vi "CRDS_Host_Test.vi"() -> ()   [LabVIEW 2012]
doc: "Host interface for communication with CRD and PAS. This application currently must be running before the servers (PAS and CRD chassis) are running). At startup, the host will poll the LAN for a UDP connection to each instrument, pinging on port 5555. The acquisition loop will configure the FP and then move into a waiting state where it is polling for a connection on TCP/IP using the STM Connection Manager. When one of the instruments responds to the host, a new TCP connection will be opened on port 5556 and added to the connection manager. Seeing the connection, this VI will move from a wait state to the acquisition state where connections will be monitored. \n\nDuring the acquisition state, the host will handle messages sent via TCP/IP from the instruments. A queued state machine will determine how the data packets sent from the different instruments is handled."
uses:
  Controls/rt_host_state.ctl
  <vilib>/Utility/Variable/NI_VariableUtilities.lvlib
  Controls/pasLasCtl.ctl
  Reusable/PAS/Main/Controls/Laser Modulation.ctl
  Utilities/FPGA/Controls/FPGAConfig.ctl
panel:
  in  "swDispl":T1
  in  "tabCtl":T2(tab)=enum."PAS Ctl"
  out "P":cluster{"hum":sgl, "dry":sgl, "ref":sgl} caption="Pressure (mb)" {"ref" format="%#.2f"; "dry" format="%#.2f"; "hum" format="%#.2f"}
  out "vaisalaData":T3 caption="Vaisala Data" {"ref"."TRH" format="%#.2f"; "ref"."RH" format="%#.2f"; "dry"."TRH" format="%#_2f"; "dry"."RH" format="%#_2f"; "hum"."TRH" format="%#_2g"; "hum"."RH" format="%#_2g"}
  out "alctData":T4 caption="Alicat Data" {"purge"."P" format="%.2f"; "purge"."T" format="%.2f"; "purge"."Q" format="%.2f"; "ref"."P" format="%.2f"; "ref"."T" format="%.2f"; "ref"."Q" format="%.2f"; "dry"."P" format="%.2f"; "dry"."T" format="%.2f"; "dry"."Q" format="%.2f"; "hum"."P" format="%.2f"; "hum"."T" format="%.2f"; "hum"."Q" format="%.2f"}
  in  "Laser Controls":cluster{"f (Hz)":dbl, "Duty Cycle (%)":dbl}
  in  "crdHeaterSP":cluster{"T1":sgl, "T2":sgl} caption="Heater Setpoints (degC)" {"T2" format="%.1f"; "T1" format="%.1f"}
  out "crdHeater":cluster{"T1":sgl, "T2":sgl} caption="Heater Temperature (degC)" {"T2" format="%.1g"; "T1" format="%.1g"}
  in  "crdFlows":T5 caption="Flow Rate Setpoints (LPM)" {"purge" max=5 format="%.2f"; "ref" max=5 format="%.2f"; "dry" max=5 format="%.2f"; "hum" max=5 format="%.2f"}
  out "crdTtec":sgl caption="TEC Temperature\n(degC)" format="%#.1f"
  in  "pasTECEn":T6 caption="Enable TECs"
  in  "pasTcell":T7 caption="Temperature \n (degC)"
  in  "pasFlows":T8 caption="Flow Rate Setpoint (LPM)" {"Cell 5" min=0.0 max=5.0; "Cell 4" min=0.0 max=5.0; "Cell 3" min=0.0 max=5.0; "Cell 2" min=0.0 max=5.0; "Cell 1" min=0.0 max=5.0}
  in  "pasLasCtl":T9={"Laser Output"={"Span"={"ch 1"=1.5, "ch 2"=1.5, "ch 3"=5.0, "ch 4"=5.0, "ch 5"=5.0}, "mod"={"ch 1"=enum."Sine", "ch 2"=enum."Sine", "ch 3"=enum."Sine", "ch 4"=enum."Sine", "ch 5"=enum."Sine"}}, "f0"={"Cell 1"=1360.2863, "Cell 2"=1358.2849, "Cell 3"=1355.6958, "Cell 4"=1355.4038, "Cell 5"=1352.1854}, "drive"=FALSE, "lasSysPow"=TRUE, "Speake Voltage"=0.0} caption="Laser Control" {"Laser Output"."Span"."ch 5" min=0 max=20; "Laser Output"."Span"."ch 4" min=0 max=20; "Laser Output"."Span"."ch 3" min=0 max=20; "Laser Output"."Span"."ch 2" min=0 max=20; "Laser Output"."Span"."ch 1" min=0 max=20; "f0"."Cell 1" format="%#.2f"; "f0"."Cell 2" format="%#.2f"; "f0"."Cell 3" format="%#.2f"; "f0"."Cell 4" format="%#.2f"; "f0"."Cell 5" format="%#.2f"}
  in  "DCPS":bool caption="DC Power Supply"
  in  "pasTteSP":sgl caption="TEC Temperature \nSetpoint (degC)" format="%#.2f"
  out "crdData":bool caption="CRD Data"
  out "pasErr":bool caption="PAS Error"
  out "pasCfg":bool caption="PAS Config"
  out "crdError":bool caption="CRDS Error"
  out "servAct":bool caption="Server Active"
  # "CRD Controls"
  # "CRD Controller Data"
  # "PAS Controls"
  # "PAS Housekeeping Data"
  # "TEC Temperature Control"
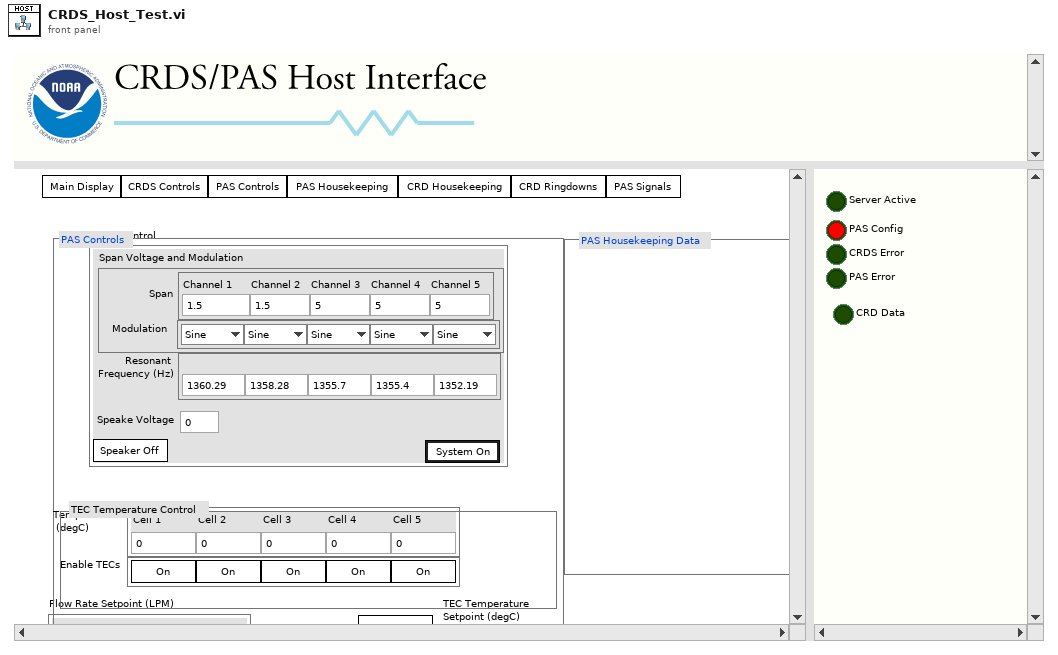
[diagram p1: front panel]
types:
  T1 = cluster{"mDispl":bool, "crdCtl":bool, "pasCtl":bool, "pasHK":bool, "crdHK":bool, "crdRD":bool, "pasSig":bool}
  T2 = enum32{"main", "CRDCtl", "PAS Ctl", "pasHK", "crdHK", "crdRD", "pasSig"}
  T3 = cluster{"hum":cluster{"RH":sgl, "TRH":sgl}, "dry":cluster{"RH":sgl, "TRH":sgl}, "ref":cluster{"RH":sgl, "TRH":sgl}}
  T4 = cluster{"hum":cluster{"Q":sgl, "T":sgl, "P":sgl}, "dry":cluster{"Q":sgl, "T":sgl, "P":sgl}, "ref":cluster{"Q":sgl, "T":sgl, "P":sgl}, "purge":cluster{"Q":sgl, "T":sgl, "P":sgl}}
  T5 = cluster{"hum":sgl, "dry":sgl, "ref":sgl, "purge":sgl}
  T6 = cluster{"Cell 1":bool, "Cell 2":bool, "Cell 3":bool, "Cell 4":bool, "Cell 5":bool}
  T7 = cluster{"Cell 1":sgl, "Cell 2":sgl, "Cell 3":sgl, "Cell 4":sgl, "Cell 5":sgl}
  T8 = cluster{"Cell 1":dbl, "Cell 2":dbl, "Cell 3":dbl, "Cell 4":dbl, "Cell 5":dbl}
  T9 = typedef "pasLasCtl.ctl" = cluster{"Laser Output":T10, "f0":cluster{"Cell 1":sgl, "Cell 2":sgl, "Cell 3":sgl, "Cell 4":sgl, "Cell 5":sgl}, "drive":bool, "lasSysPow":bool, "Speake Voltage":dbl}
  T10 = typedef "FPGAConfig.ctl" = cluster{"Span":cluster{"ch 1":sgl, "ch 2":sgl, "ch 3":sgl, "ch 4":sgl, "ch 5":sgl}, "mod":cluster{"ch 1":T11, "ch 2":T11, "ch 3":T11, "ch 4":T11, "ch 5":T11}}
  T11 = typedef "Laser Modulation.ctl" = enum8{"Sine", "Square"}
  T12 = typedef "rt_host_state.ctl" = enum16{"Config", "CRD Comm", "PAS Comm", "Wait", "Quit"}
  T13 = cluster{"c 1":bool, "c 2":bool, "c 3":bool, "c 4":bool, "c 5":bool}
  T14 = cluster{"[0]":bool, "[1]":bool, "[2]":bool, "[3]":bool, "[4]":bool, "[5]":bool, "[6]":bool}
  T15 = enum32{"invalid app kind", "Development System", "Run Time System", "Student Edition", "Embedded LabVIEW", "Evaluation", "Custom"}
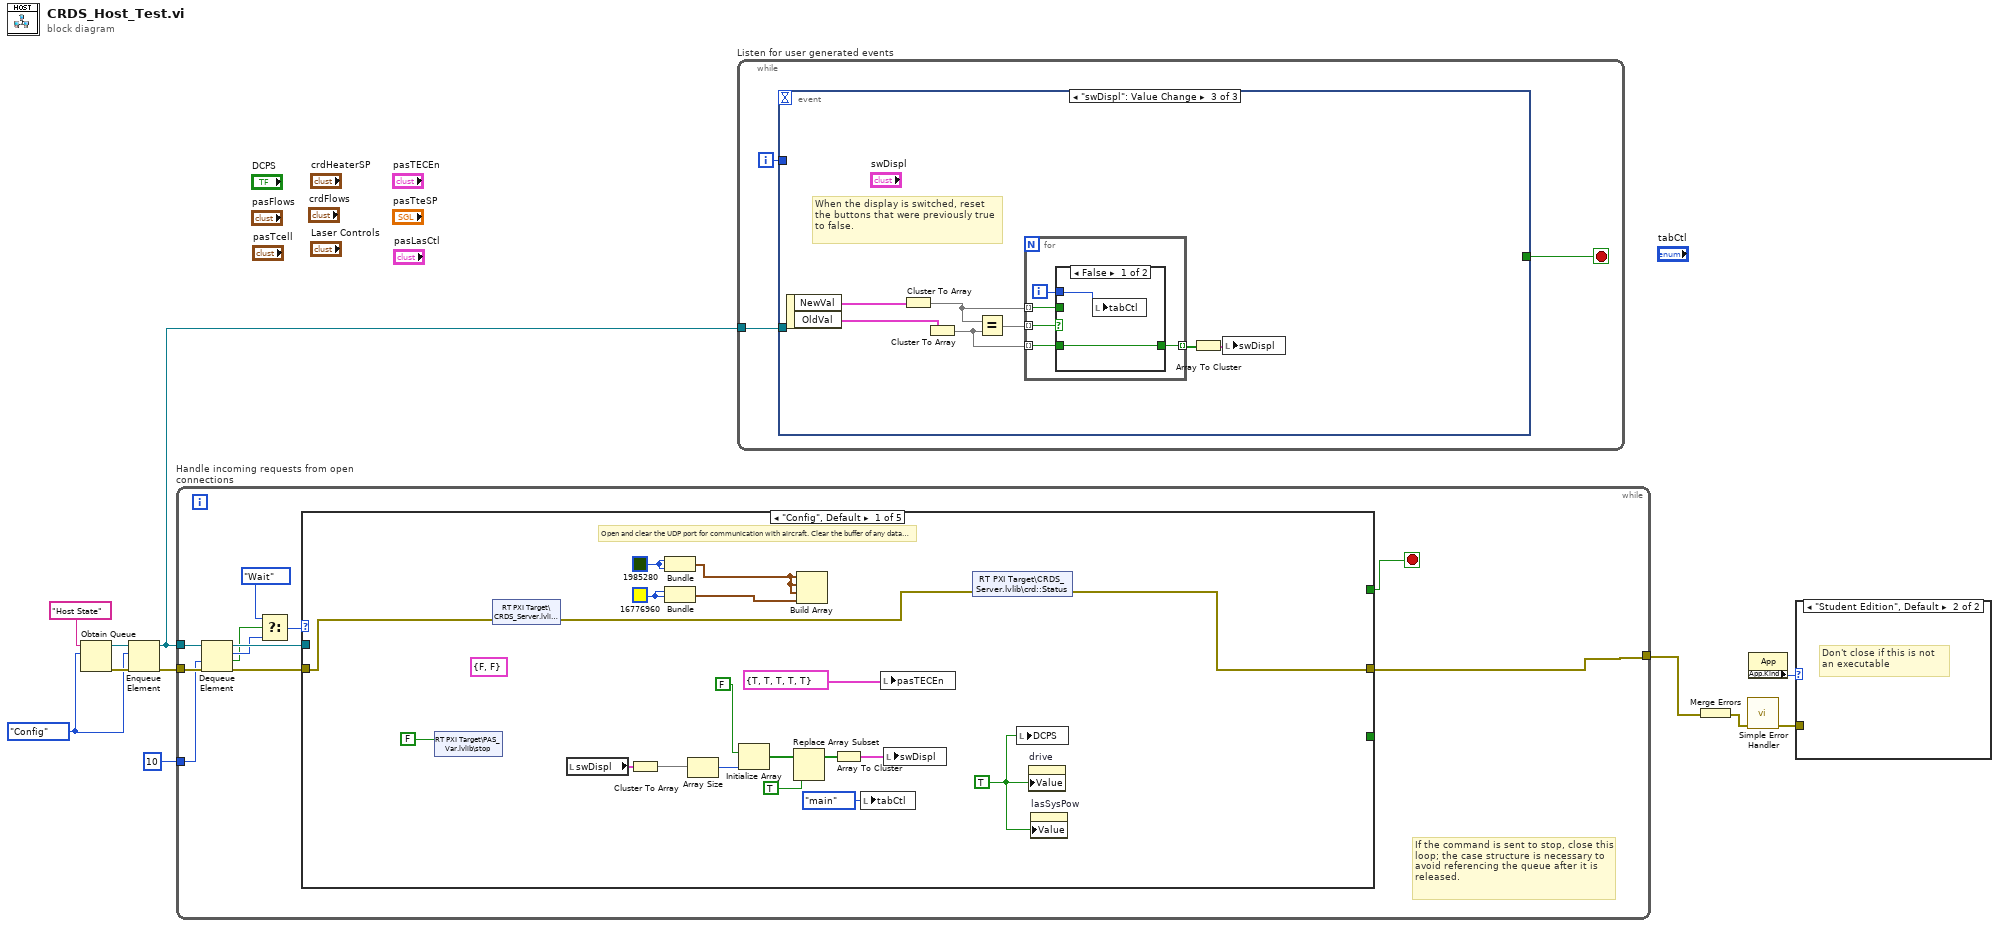
[diagram p0: block diagram]
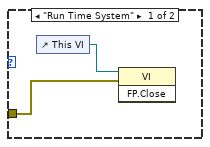
[diagram p2: hidden frame]
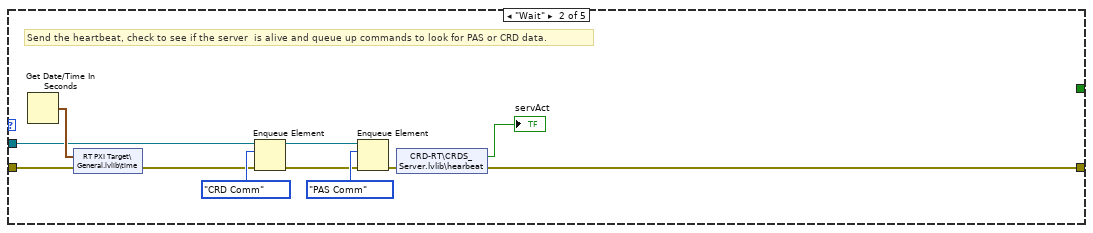
[diagram p3: hidden frame]
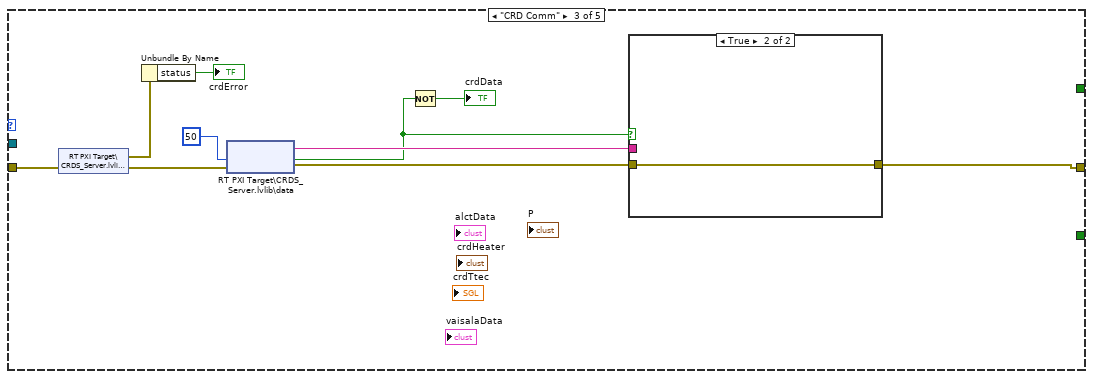
[diagram p4: hidden frame]
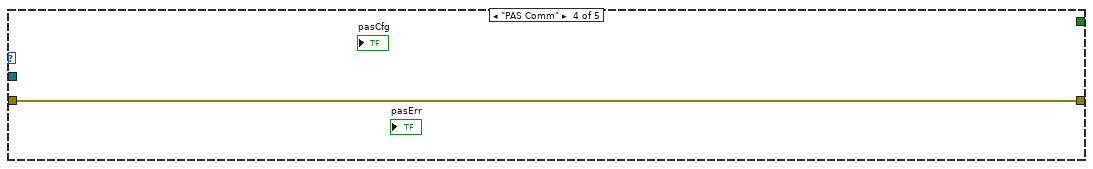
[diagram p6: hidden frame]
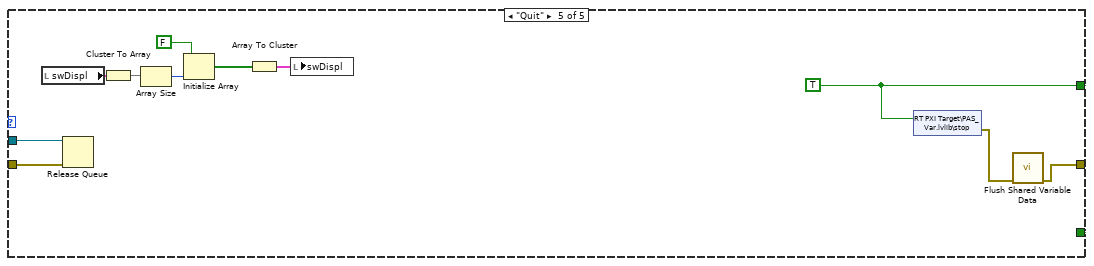
[diagram p7: hidden frame]
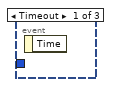
[diagram p8: hidden frame]
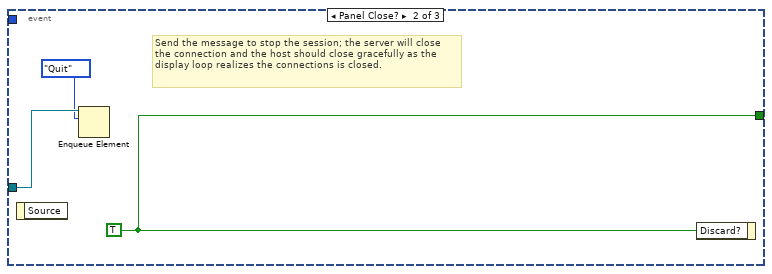
[diagram p9: hidden frame]
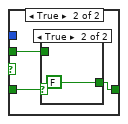
[diagram p10: hidden frame]
diagram:
  w7 = rt_host_state."Config" ("Host_State")
  n1 = Obtain Queue(name (unnamed)="Host State", element data type=w7) -> (queue out=w10:refnum<queue>, error out=w9:errorcluster)  [unwired: 3 in, 1 out]
  n2 = Enqueue Element(queue=w10, element=w7, error in (no error)=w9) -> (queue out=w1:refnum<queue>, error out=w8:errorcluster)  [unwired: 1 in, 1 out]
  n3 = while "Handle incoming requests from open connections" {
    tunnel: w1 -> [w22]
    tunnel: w8 -> [w20]
    tunnel: [w12] -> w6
    tunnel: 10 ("timeout in ms (-1)") -> [w13]
    stop <- w18 stop-if-true
    # "If the command is sent to stop, close this loop; the case structure is necessary to avoid referencing the queue after it is released."
    n4 = Dequeue Element(queue=w22, timeout in ms (-1)=w13, error in (no error)=w20) -> (queue out=w21:refnum<queue>, element=w17:T12, timed out?=w15:bool, error out=w19:errorcluster)
    n5 = Select(t=rt_host_state."Wait", s=w15, f=w17) -> (s? t:f=w14:T12)
    n6 = case shown="\"Config\", Default" w14 {
      tunnel: w19 -> [w24 w51 w58 w65 w69]
      tunnel: w21 -> [_ w50 _ _ w76]
      tunnel: [_ _ _ _ w68] -> w18
      tunnel: [_ _ _ _ w68] -> _
      tunnel: [w25 w49 w59 w65 w66] -> w12
      frame "Config", Default {
        w27 = TRUE ("Value")
        w29 = u32 16776960
        w28 = u32 1985280
        (unwired) cluster{"CRD":bool, "PAS":bool} {"CRD"=FALSE, "PAS"=FALSE} ("filtSwitch")
        # "Open and clear the UDP port for communication with aircraft. Clear the buffer of any data currently on line."
        n7 = shared-variable "RT PXI Target\\PAS_Var.lvlib\\stop"(FALSE ("stop")) -> ()  [unwired: 1 in, 1 out]
        n8 = shared-variable "RT PXI Target\\CRDS_Server.lvlib\\data"(error in=w24) -> (error out=w23:errorcluster)  [unwired: 1 out]
        n9 = local read "swDispl"() -> (w41:T1)
        n10 = Cluster To Array(cluster=w41) -> (array=w40:bool[])
        n11 = Bundle(w28, w28) -> (w31:cluster{u32, u32})  [unwired: 1 in]
        n12 = Bundle(w29, w29) -> (w30:cluster{u32, u32})  [unwired: 1 in]
        n13 = Array Size(array=w40) -> (size(s)=w39:i32)
        n14 = Initialize Array(FALSE, w39) -> (w38:bool[])
        n15 = Replace Array Subset(array=w38, new element=TRUE ("new element/subarray")) -> (w36:bool[])  [unwired: 1 in]
        n16 = Build Array(w31, w31, w31, w30) -> ()  [unwired: 1 out]
        n17 = Array To Cluster(array=w36) -> (cluster=w35:T14)
        n18 = local write "tabCtl"(T2."main" ("tabCtl")) -> ()
        n19 = local write "pasTECEn"(T13 {"c 1"=TRUE, "c 2"=TRUE, "c 3"=TRUE, "c 4"=TRUE, "c 5"=TRUE} ("pasTECEn")) -> ()
        n20 = local write "swDispl"(w35) -> ()
        n21 = shared-variable "RT PXI Target\\CRDS_Server.lvlib\\crd::Status"(error in=w23) -> (error out=w25:errorcluster)  [unwired: 1 out]
        n22 = local write "DCPS"(w27) -> ()
        n23 = property on="drive" class="Bool (strict)"("Value"=w27) -> ()  [unwired: 2 in, 2 out]
        n24 = property on="lasSysPow" class="Bool (strict)"("Value"=w27) -> ()  [unwired: 2 in, 2 out]
      }
      frame "Wait" {
        # "Send the heartbeat, check to see if the server  is alive and queue up commands to look for PAS or CRD data."
        n25 = Get Date/Time In Seconds() -> (seconds since 1Jan1904=w52:timestamp)
        n26 = shared-variable "RT PXI Target\\General.lvlib\\time"(w52, error in=w51) -> (error out=w42:errorcluster)
        n27 = Enqueue Element(queue=w50, element=rt_host_state."CRD Comm", error in (no error)=w42) -> (queue out=w47:refnum<queue>, error out=w43:errorcluster)  [unwired: 1 in, 1 out]
        n28 = Enqueue Element(queue=w47, element=rt_host_state."PAS Comm", error in (no error)=w43) -> (error out=w46:errorcluster)  [unwired: 1 in, 2 out]
        n29 = shared-variable "CRD-RT\\CRDS_Server.lvlib\\hearbeat"(error in=w46) -> (→"servAct":bool, error out=w49:errorcluster)
      }
      frame "CRD Comm" {
        n30 = shared-variable "RT PXI Target\\CRDS_Server.lvlib\\error"(error in=w58) -> (w56:errorcluster, error out=w57:errorcluster)
        n31 = Unbundle By Name(w56) -> ("status"=→"crdError":bool)
        n32 = shared-variable "RT PXI Target\\CRDS_Server.lvlib\\data"(error in=w57, 50 ("ms timeout (0)")) -> (w62:string, error out=w61:errorcluster, w54:bool)
        n33 = Not(x=w54) -> (.not. x?=→"crdData":bool)
        n34 = case shown="True" w54 {
          tunnel: w62 -> [_ _]
          tunnel: w61 -> [w63 w64]
          tunnel: [w63 w64] -> w59
          frame False {
          }
          frame True {
          }
        }
      }
      frame "PAS Comm" {
      }
      frame "Quit" {
        w68 = TRUE
        n35 = local read "swDispl"() -> (w75:T1)
        n36 = Release Queue(queue=w76, error in (no error)=w69) -> ()  [unwired: 1 in, 3 out]
        n37 = Cluster To Array(cluster=w75) -> (array=w74:bool[])
        n38 = Array Size(array=w74) -> (size(s)=w73:i32)
        n39 = Initialize Array(FALSE, w73) -> (w71:bool[])
        n40 = Array To Cluster(array=w71) -> (cluster=w70:T14)
        n41 = local write "swDispl"(w70) -> ()
        n42 = shared-variable "RT PXI Target\\PAS_Var.lvlib\\stop"(w68) -> (error out=w67:errorcluster)  [unwired: 1 in]
        n43 = call <vilib>:"Flush Shared Variable Data.vi"("error in (no error)"=w67) -> ("error out"=w66:errorcluster)  [unwired: 10 in]
      }
    }
  }
  n44 = while "Listen for user generated events" {
    tunnel: w1 -> [w77]
    i -> [w79]
    stop <- w78 stop-if-true
    n45 = event shown="[2] \"swDispl\": Value Change" {
      selector: _ -> [_ _ _]
      dyn-events: _ -> [_ _ _]
      timeout: _ -> [_ _ _]
      tunnel: [_ w82 _] -> w78
      tunnel: w79 -> [_ _ _]
      tunnel: w77 -> [_ w81 _]
      event Timeout {
        n46 = event-data() -> ()  [unwired: 1 in, 1 out]
      }
      event Panel Close? {
        w82 = TRUE ("Discard?")
        # "Send the message to stop the session; the server will close the connection and the host should close gracefully as the display loop realizes the connections is closed."
        n47 = event-data() -> ()  [unwired: 1 in, 1 out]
        n48 = Enqueue Element(queue=w81, element=rt_host_state."Quit") -> ()  [unwired: 2 in, 3 out]
        n49 = event-data("Discard?"=w82) -> ()  [unwired: 1 in, 1 out]
      }
      event "swDispl": Value Change {
        # "When the display is switched, reset the buttons that were previously true to false."
        n50 = event-data() -> ("NewVal"=w88:T1, "OldVal"=w89:T1)  [unwired: 1 in]
        n51 = Cluster To Array(cluster=w88) -> (array=w85:bool[])
        n52 = Cluster To Array(cluster=w89) -> (array=w86:bool[])
        n53 = Equal?(x=w85, y=w86) -> (x = y?=w87:bool[])
        n54 = for {
          tunnel: w87 -> [w94] mode=indexing
          tunnel: w86 -> [w93] mode=indexing
          tunnel: [w92] -> w84 mode=indexing
          tunnel: w85 -> [w91] mode=indexing
          i -> [w90]
          n55 = case shown="False" w94 {
            tunnel: w93 -> [_ w99]
            tunnel: [w96 w98] -> w92
            tunnel: w91 -> [w96 w97]
            tunnel: w90 -> [w95 _]
            frame False {
              n56 = local write "tabCtl"(w95) -> ()
            }
            frame True {
              n57 = case shown="True" w99 {
                tunnel: [w100 FALSE] -> w98
                tunnel: w97 -> [w100 _]
                frame False {
                }
                frame True {
                }
              }
            }
          }
        }
        n58 = Array To Cluster(array=w84) -> (cluster=w83:T14)
        n59 = local write "swDispl"(w83) -> ()
      }
    }
  }
  n60 = Merge Errors(w6) -> (w5:errorcluster)
  n61 = call <vilib>:"Simple Error Handler.vi"("error in (no error)"=w5) -> ("error out"=w3:errorcluster)  [unwired: 4 in, 4 out]
  n62 = property class="App"() -> ("App.Kind"=w2:T15)  [unwired: 2 in, 2 out]
  n63 = case shown="\"Student Edition\", Default" w2 {
    tunnel: w3 -> [w102 _]
    frame "Run Time System" {
      n64 = control-ref of="This VI"() -> (w103:refnum<vi>)
      n65 = invoke class="VI" method="FP.Close"(reference=w103, error in=w102) -> ()  [unwired: 1 in, 3 out]
    }
    frame "Student Edition", Default {
      # "Don't close if this is not \nan executable"
    }
  }
